vi "字串.vi"() -> ()   [LabVIEW 2021]
panel:
  out "String":string="歡迎"
  in  "輸入帳號":string
  out "結果":string
  in  "存入":dbl
  out "正確":bool
  out "密碼確認":string
  in  "輸入密碼":string
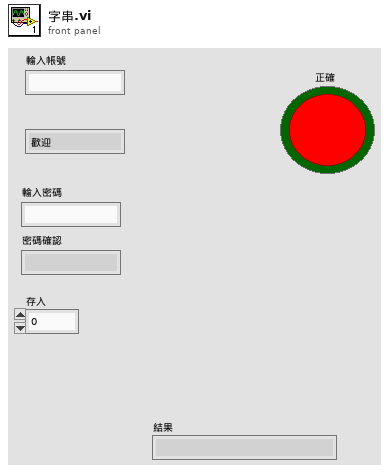
[diagram p1: front panel]
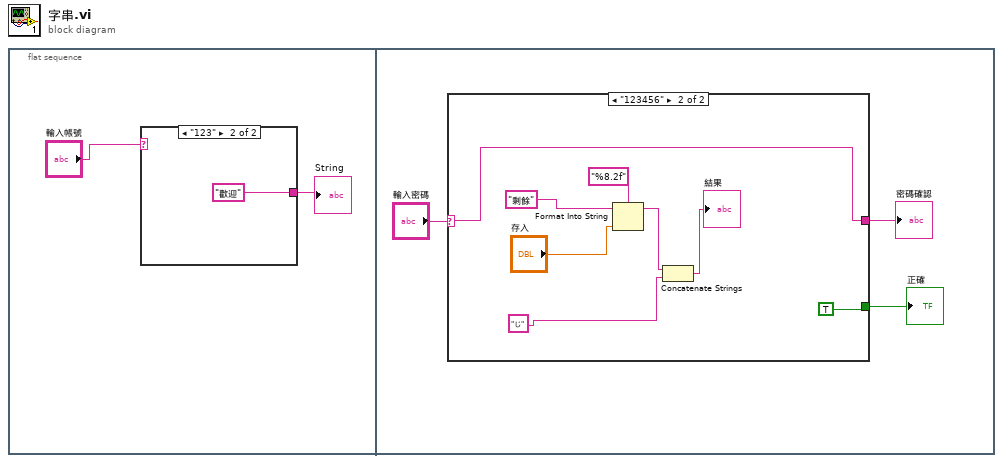
[diagram p0: block diagram]
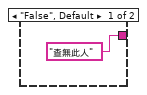
[diagram p2: hidden frame]
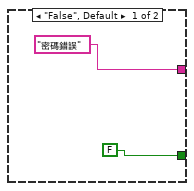
[diagram p3: hidden frame]
diagram:
  n1 = flat-sequence {
    frame #0 {
      n2 = case shown="\"123\"" "輸入帳號" {
        tunnel: ["查無此人" "歡迎"] -> w1
        frame "False", Default {
        }
        frame "123" {
        }
      }
      "String" <- w1
    }
    frame #1 {
      n3 = case shown="\"123456\"" "輸入密碼" {
        selector: "輸入密碼" -> [_ w14]
        tunnel: ["密碼錯誤" w14] -> w6
        tunnel: [FALSE TRUE] -> w7
        frame "False", Default {
        }
        frame "123456" {
          n4 = Format Into String(format string="%8.2f", initial string="剩餘", "存入") -> (resulting string=w16:string)  [unwired: 1 in, 1 out]
          n5 = Concatenate Strings(w16, "じ") -> (→"結果":string)
        }
      }
      "密碼確認" <- w6
      "正確" <- w7
    }
  }
